vi "fit 3 section stuckbead.vi"(0 "X=T; Y=F":bool) -> (1 "bead position out (nm)":dbl[](array[numeric]), 2 "best fit position out":dbl[](array[numeric]), 3 "(1+2+3) stuckbead-scan coefficient":T1 {"(3)stuckbead-scan coefficient" min=0.0 max=127.0 format="%#.2f"; "(2)stuckbead-scan coefficient" min=0.0 max=127.0 format="%#.2f"; "(1)stuckbead-scan coefficient" min=0.0 max=127.0 format="%#.2f"}, 4 "Calib-stage position (um)":dbl[](array[numeric]), 5 "Calib-QPD scan (V)":dbl[](array[numeric]))   [LabVIEW 2014]
uses:
  (1+2+3)fit stuckbead coefficient.ctl
  <vilib>/Utility/file.llb/Read From Spreadsheet File (DBL).vi
  <vilib>/Analysis/polynomials.llb/Scalar Polynomial Evaluation (DBL).vi
  <vilib>/Analysis/NI_AALPro.lvlib
panel:
  out "center of position (um)":dbl
  out "P(a)":dbl
  in  "a":dbl
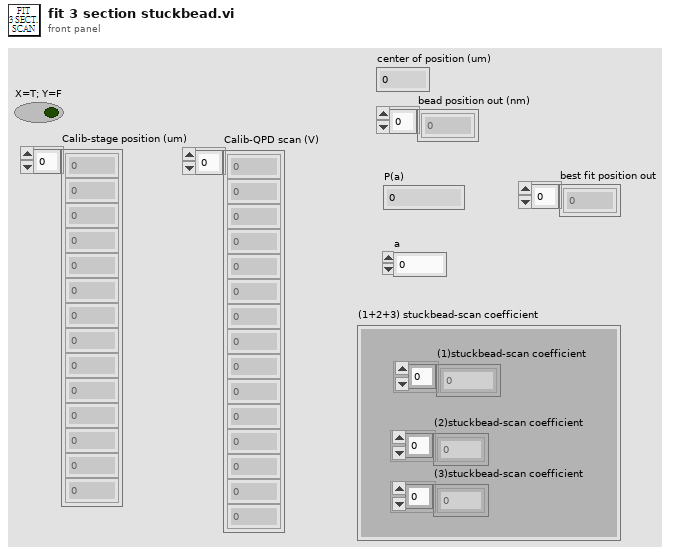
[diagram p1: front panel]
types:
  T1 = typedef "(1+2+3)fit stuckbead coefficient.ctl" = cluster{"(1)stuckbead-scan coefficient ":dbl[], "(2)stuckbead-scan coefficient ":dbl[], "(3)stuckbead-scan coefficient":dbl[]}
  T2 = cluster{"Polynomial Coefficients":dbl[], "Polynomial Coefficients":dbl[], "Polynomial Coefficients":dbl[]}
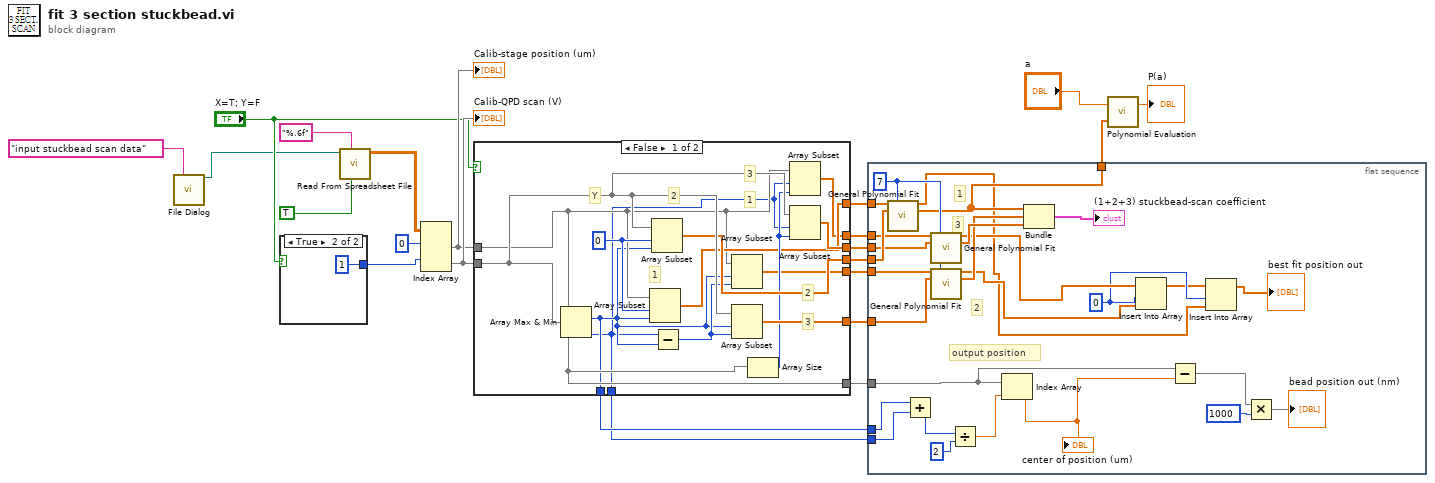
[diagram p0: block diagram]
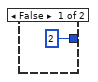
[diagram p2: hidden frame]
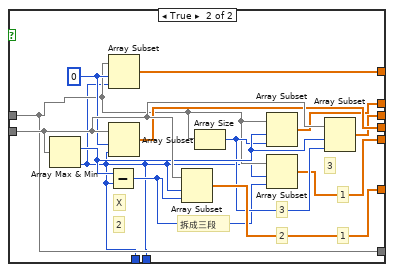
[diagram p3: hidden frame]
diagram:
  n1 = call "File Dialog"("prompt"="input stuckbead scan data") -> ("selected path"=w4:path)  [unwired: 11 in, 3 out]
  n2 = case shown="True" "X=T; Y=F" {
    tunnel: [2 1] -> w9
    frame False {
    }
    frame True {
    }
  }
  n3 = call-poly <vilib>:"Read From Spreadsheet File.vi"("transpose (no:F)"=TRUE, "format (%.3f)"="%.6f", "file path (dialog if empty)"=w4) -> ("all rows"=w14:dbl[][])  [unwired: 4 in, 4 out]
  n4 = Index Array(array=w14, index (row) #1=0 ("index (row)"), index (row) #2=w9) -> (element #1=w11:dbl[], element #2=w12:dbl[])  [unwired: 2 in]
  "Calib-QPD scan (V)" <- w12
  "Calib-stage position (um)" <- w11
  n5 = case shown="False" "X=T; Y=F" {
    tunnel: w12 -> [w37 w50]
    tunnel: [w36 w49] -> w21
    tunnel: [w35 w48] -> w22
    tunnel: [w34 w47] -> w20
    tunnel: w11 -> [w27 w39]
    tunnel: [w30 w42] -> w19
    tunnel: [w29 w41] -> w18
    tunnel: [w28 w40] -> w17
    tunnel: [w27 w39] -> w3
    tunnel: [w26 w38] -> w2
    tunnel: [w25 w38] -> w1
    frame False {
      w33 = 0 ("index")
      # "2"
      # "3"
      # "1"
      # "Y"
      # "3"
      # "2"
      # "1"
      n6 = Array Max & Min(array=w37) -> (max index (indices)=w26:i32, min index (indices)=w25:i32)  [unwired: 2 out]
      n7 = Array Subset(array=w27, index=w33, length=w26) -> (w30:dbl[])
      n8 = Array Subset(array=w37, index=w33, length=w26) -> (w36:dbl[])
      n9 = Subtract(x=w25, y=w26) -> (x-y=w31:i32)
      n10 = Array Subset(array=w27, index=w26, length=w31) -> (w29:dbl[])
      n11 = Array Subset(array=w37, index=w26, length=w31) -> (w35:dbl[])
      n12 = Array Size(array=w27) -> (size(s)=w32:i32)
      n13 = Array Subset(array=w27, index=w25, length=w32) -> (w28:dbl[])
      n14 = Array Subset(array=w37, index=w25, length=w32) -> (w34:dbl[])
    }
    frame True {
      w46 = 0 ("index")
      # "3"
      # "2"
      # "1"
      # "拆成三段"
      # "X"
      # "3"
      # "2"
      # "1"
      n15 = Array Max & Min(array=w50) -> (max index (indices)=w45:i32, min index (indices)=w38:i32)  [unwired: 2 out]
      n16 = Subtract(x=w45, y=w38) -> (x-y=w43:i32)
      n17 = Array Subset(array=w39, index=w46, length=w38) -> (w42:dbl[])
      n18 = Array Subset(array=w50, index=w46, length=w38) -> (w49:dbl[])
      n19 = Array Subset(array=w50, index=w38, length=w43) -> (w48:dbl[])
      n20 = Array Size(array=w39) -> (size(s)=w44:i32)
      n21 = Array Subset(array=w39, index=w45, length=w44) -> (w40:dbl[])
      n22 = Array Subset(array=w39, index=w38, length=w43) -> (w41:dbl[])
      n23 = Array Subset(array=w50, index=w45, length=w44) -> (w47:dbl[])
    }
  }
  n24 = flat-sequence {
    tunnel: w22 -> [w77]
    tunnel: w21 -> [w76]
    tunnel: w20 -> [w75]
    tunnel: w19 -> [w74]
    tunnel: w18 -> [w73]
    tunnel: w17 -> [w72]
    tunnel: [w67] -> w8
    tunnel: w3 -> [w55]
    tunnel: w2 -> [w59]
    tunnel: w1 -> [w58]
    frame #0 {
      w64 = 0 ("index")
      w68 = 7 ("polynomial order")
      # "output position"
      # "3"
      # "2"
      # "1"
      n25 = call <vilib>:"General Polynomial Fit.vi"("Y"=w74, "polynomial order"=w68, "X"=w76) -> ("Best Polynomial Fit"=w62:dbl[], "Polynomial Coefficients"=w67:dbl[])  [unwired: 9 in, 2 out]
      n26 = Add(x=w59, y=w58) -> (x+y=w60:i32)
      n27 = call <vilib>:"General Polynomial Fit.vi"("Y"=w72, "polynomial order"=w68, "X"=w75) -> ("Best Polynomial Fit"=w66:dbl[], "Polynomial Coefficients"=w71:dbl[])  [unwired: 9 in, 2 out]
      n28 = call <vilib>:"General Polynomial Fit.vi"("Y"=w73, "polynomial order"=w68, "X"=w77) -> ("Best Polynomial Fit"=w65:dbl[], "Polynomial Coefficients"=w69:dbl[])  [unwired: 9 in, 2 out]
      n29 = Divide(x=w60, y=2) -> (x/y=w56:dbl)
      n30 = Index Array(array=w55, index=w56) -> (element=w54:dbl)
      "center of position (um)" <- w54
      n31 = Bundle("Polynomial Coefficients"=w67, "Polynomial Coefficients"=w69, "Polynomial Coefficients"=w71) -> (→"(1+2+3) stuckbead-scan coefficient":T2)  [unwired: 1 in]
      n32 = Insert Into Array(array=w66, index=w64, new element=w65) -> (w63:dbl[])
      n33 = Subtract(x=w55, y=w54) -> (x-y=w53:dbl[])
      n34 = Insert Into Array(array=w63, index=w64, new element=w62) -> (→"best fit position out":dbl[])
      n35 = Multiply(x=w53, y=1000) -> (x*y=→"bead position out (nm)":dbl[])
    }
  }
  n36 = call-poly <vilib>:"Polynomial Evaluation.vi"("P(x)"=w8, "a"="a") -> ("P(a)"=→"P(a)":dbl)  [unwired: 1 out]
